vi "slide tab.vi"(0 "Tab Ref In":refnum<vi>, 5 "slide (right)":i32, 7 "slide (down)":i32, 9 "enlarge (width)":i32, 11 "enlarge (height)":i32, 12 "pixel shift":i32=10) -> ()   [LabVIEW 2017]
doc: "SciScan 1.2 160622"
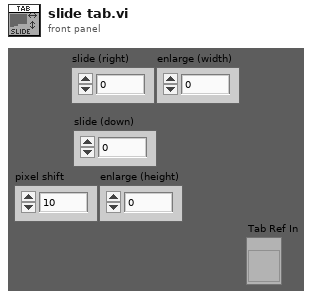
[diagram p1: front panel]
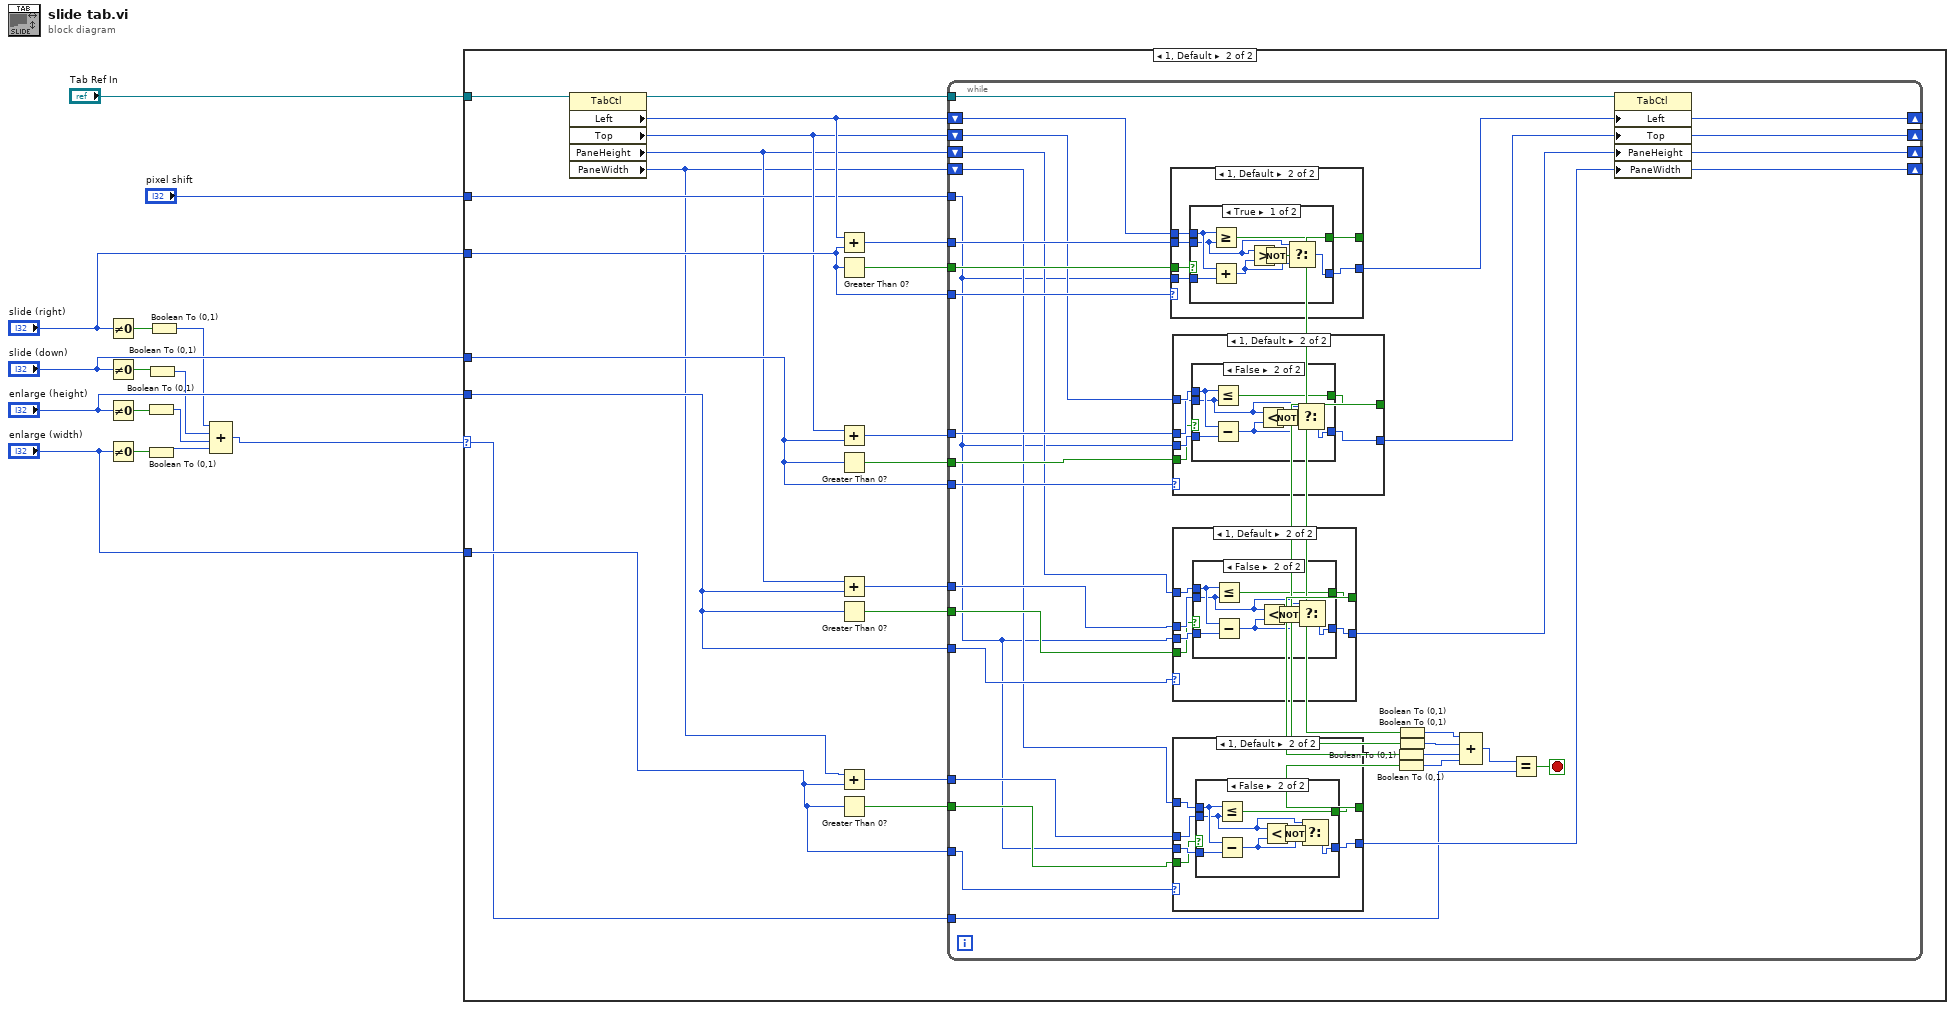
[diagram p0: block diagram]
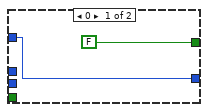
[diagram p3: hidden frame]
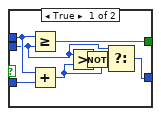
[diagram p4: hidden frame]
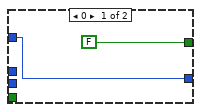
[diagram p5: hidden frame]
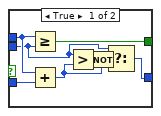
[diagram p6: hidden frame]
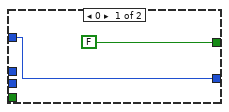
[diagram p7: hidden frame]
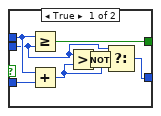
[diagram p8: hidden frame]
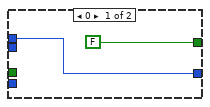
[diagram p9: hidden frame]
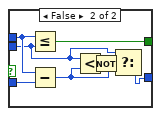
[diagram p10: hidden frame]
diagram:
  n1 = Not Equal To 0?(x="slide (right)") -> (x != 0?=w9:bool)
  n2 = Not Equal To 0?(x="slide (down)") -> (x != 0?=w8:bool)
  n3 = Not Equal To 0?(x="enlarge (height)") -> (x != 0?=w7:bool)
  n4 = Not Equal To 0?(x="enlarge (width)") -> (x != 0?=w6:bool)
  n5 = Boolean To (0,1)(Boolean=w7) -> (0, 1=w3:i16)
  n6 = Boolean To (0,1)(Boolean=w6) -> (0, 1=w2:i16)
  n7 = Boolean To (0,1)(Boolean=w8) -> (0, 1=w4:i16)
  n8 = Boolean To (0,1)(Boolean=w9) -> (0, 1=w5:i16)
  n9 = Compound Arithmetic op=ADD(w5, w4, w3, w2) -> (w1:i16)
  n10 = case shown="1, Default" w1 {
    selector: w1 -> [_ w16]
    tunnel: "Tab Ref In" -> [_ w35]
    tunnel: "slide (right)" -> [_ w30]
    tunnel: "slide (down)" -> [_ w28]
    tunnel: "enlarge (height)" -> [_ w24]
    tunnel: "enlarge (width)" -> [_ w23]
    tunnel: "pixel shift" -> [_ w25]
    frame 0 {
    }
    frame 1, Default {
      n11 = property class="TabCtl"(reference=w35) -> (reference out=w34:refnum<vi>, "Left"=w27:i32, "Top"=w26:i32, "PaneHeight"=w20:u32, "PaneWidth"=w17:u32)  [unwired: 1 in, 1 out]
      n12 = Add(x=w27, y=w30) -> (x+y=w33:i32)
      n13 = Greater Than 0?(x=w30) -> (x > 0?=w31:bool)
      n14 = Add(x=w26, y=w28) -> (x+y=w32:i32)
      n15 = Greater Than 0?(x=w28) -> (x > 0?=w29:bool)
      n16 = Add(x=w20, y=w24) -> (x+y=w21:u32)
      n17 = Greater Than 0?(x=w24) -> (x > 0?=w22:bool)
      n18 = Add(x=w17, y=w23) -> (x+y=w18:u32)
      n19 = Greater Than 0?(x=w23) -> (x > 0?=w19:bool)
      n20 = while {
        tunnel: w34 -> [w62]
        tunnel: w25 -> [w49]
        tunnel: w33 -> [w68]
        tunnel: w32 -> [w67]
        tunnel: w31 -> [w66]
        tunnel: w30 -> [w65]
        tunnel: w29 -> [w64]
        tunnel: w28 -> [w63]
        shift-right: [w59] -> _
        shift-left: w27 -> [w60]
        shift-right: [w58] -> _
        shift-left: w26 -> [w61]
        shift-right: [w48] -> _
        shift-left: w20 -> [w54]
        shift-right: [w47] -> _
        shift-left: w17 -> [w50]
        tunnel: w24 -> [w56]
        tunnel: w23 -> [w53]
        tunnel: w22 -> [w57]
        tunnel: w21 -> [w55]
        tunnel: w19 -> [w52]
        tunnel: w18 -> [w51]
        tunnel: w16 -> [w37]
        stop <- w36 stop-if-true
        n21 = case shown="1, Default" w65 {
          tunnel: [FALSE w148] -> w39
          tunnel: w60 -> [w141 w145]
          tunnel: w68 -> [_ w147]
          tunnel: w66 -> [_ w146]
          tunnel: w49 -> [_ w144]
          tunnel: [w141 w143] -> w59
          frame 0 {
          }
          frame 1, Default {
            n22 = case shown="True" w146 {
              tunnel: [w156 w164] -> w148
              tunnel: w145 -> [w155 w163]
              tunnel: w147 -> [w150 w160]
              tunnel: w144 -> [w154 w162]
              tunnel: [w151 w158] -> w143
              frame True {
                n23 = Greater Or Equal?(x=w155, y=w150) -> (x >= y?=w156:bool)
                n24 = Add(x=w155, y=w154) -> (x+y=w152:i32)
                n25 = Greater?(x=w150, y=w152) -> (0:w153:bool)
                n26 = Not(x=w153) -> (.not. x?=w149:bool)
                n27 = Select(t=w150, s=w149, f=w152) -> (s? t:f=w151:i32)
              }
              frame False {
                n28 = Less Or Equal?(x=w163, y=w160) -> (x <= y?=w164:bool)
                n29 = Subtract(x=w163, y=w162) -> (x-y=w159:i32)
                n30 = Less?(x=w160, y=w159) -> (x < y?=w161:bool)
                n31 = Not(x=w161) -> (.not. x?=w157:bool)
                n32 = Select(t=w160, s=w157, f=w159) -> (s? t:f=w158:i32)
              }
            }
          }
        }
        n33 = case shown="1, Default" w63 {
          tunnel: w61 -> [w117 w124]
          tunnel: w67 -> [_ w123]
          tunnel: w64 -> [_ w121]
          tunnel: [FALSE w120] -> w40
          tunnel: [w117 w119] -> w58
          tunnel: w49 -> [_ w122]
          frame 0 {
          }
          frame 1, Default {
            n34 = case shown="False" w121 {
              tunnel: [w132 w140] -> w120
              tunnel: w124 -> [w131 w139]
              tunnel: w123 -> [w126 w136]
              tunnel: w122 -> [w130 w138]
              tunnel: [w127 w134] -> w119
              frame True {
                n35 = Greater Or Equal?(x=w131, y=w126) -> (x >= y?=w132:bool)
                n36 = Add(x=w131, y=w130) -> (x+y=w128:i32)
                n37 = Greater?(x=w126, y=w128) -> (0:w129:bool)
                n38 = Not(x=w129) -> (.not. x?=w125:bool)
                n39 = Select(t=w126, s=w125, f=w128) -> (s? t:f=w127:i32)
              }
              frame False {
                n40 = Less Or Equal?(x=w139, y=w136) -> (x <= y?=w140:bool)
                n41 = Subtract(x=w139, y=w138) -> (x-y=w135:i32)
                n42 = Less?(x=w136, y=w135) -> (x < y?=w137:bool)
                n43 = Not(x=w137) -> (.not. x?=w133:bool)
                n44 = Select(t=w136, s=w133, f=w135) -> (s? t:f=w134:i32)
              }
            }
          }
        }
        n45 = case shown="1, Default" w56 {
          tunnel: w54 -> [w93 w100]
          tunnel: w55 -> [_ w99]
          tunnel: w57 -> [_ w97]
          tunnel: [FALSE w95] -> w41
          tunnel: [w93 w96] -> w48
          tunnel: w49 -> [_ w98]
          frame 0 {
          }
          frame 1, Default {
            n46 = case shown="False" w97 {
              tunnel: [w108 w116] -> w95
              tunnel: w100 -> [w107 w115]
              tunnel: w99 -> [w102 w112]
              tunnel: w98 -> [w106 w114]
              tunnel: [w103 w110] -> w96
              frame True {
                n47 = Greater Or Equal?(x=w107, y=w102) -> (x >= y?=w108:bool)
                n48 = Add(x=w107, y=w106) -> (x+y=w104:u32)
                n49 = Greater?(x=w102, y=w104) -> (0:w105:bool)
                n50 = Not(x=w105) -> (.not. x?=w101:bool)
                n51 = Select(t=w102, s=w101, f=w104) -> (s? t:f=w103:u32)
              }
              frame False {
                n52 = Less Or Equal?(x=w115, y=w112) -> (x <= y?=w116:bool)
                n53 = Subtract(x=w115, y=w114) -> (x-y=w111:u32)
                n54 = Less?(x=w112, y=w111) -> (x < y?=w113:bool)
                n55 = Not(x=w113) -> (.not. x?=w109:bool)
                n56 = Select(t=w112, s=w109, f=w111) -> (s? t:f=w110:u32)
              }
            }
          }
        }
        n57 = case shown="1, Default" w53 {
          tunnel: w50 -> [w69 w76]
          tunnel: w51 -> [_ w75]
          tunnel: w52 -> [_ w73]
          tunnel: [FALSE w72] -> w42
          tunnel: [w69 w71] -> w47
          tunnel: w49 -> [_ w74]
          frame 0 {
          }
          frame 1, Default {
            n58 = case shown="False" w73 {
              tunnel: [w84 w92] -> w72
              tunnel: w76 -> [w83 w91]
              tunnel: w75 -> [w78 w88]
              tunnel: w74 -> [w82 w90]
              tunnel: [w79 w86] -> w71
              frame True {
                n59 = Greater Or Equal?(x=w83, y=w78) -> (x >= y?=w84:bool)
                n60 = Add(x=w83, y=w82) -> (x+y=w80:u32)
                n61 = Greater?(x=w78, y=w80) -> (0:w81:bool)
                n62 = Not(x=w81) -> (.not. x?=w77:bool)
                n63 = Select(t=w78, s=w77, f=w80) -> (s? t:f=w79:u32)
              }
              frame False {
                n64 = Less Or Equal?(x=w91, y=w88) -> (x <= y?=w92:bool)
                n65 = Subtract(x=w91, y=w90) -> (x-y=w87:u32)
                n66 = Less?(x=w88, y=w87) -> (x < y?=w89:bool)
                n67 = Not(x=w89) -> (.not. x?=w85:bool)
                n68 = Select(t=w88, s=w85, f=w87) -> (s? t:f=w86:u32)
              }
            }
          }
        }
        n69 = Boolean To (0,1)(Boolean=w41) -> (0, 1=w45:i16)
        n70 = Boolean To (0,1)(Boolean=w42) -> (0, 1=w46:i16)
        n71 = Boolean To (0,1)(Boolean=w39) -> (0, 1=w43:i16)
        n72 = Boolean To (0,1)(Boolean=w40) -> (0, 1=w44:i16)
        n73 = Compound Arithmetic op=ADD(w43, w44, w45, w46) -> (w38:i16)
        n74 = Equal?(x=w38, y=w37) -> (x = y?=w36:bool)
        n75 = property class="TabCtl"(reference=w62, "Left"=w59, "Top"=w58, "PaneHeight"=w48, "PaneWidth"=w47) -> ()  [unwired: 1 in, 2 out]
      }
    }
  }
